vi "Save_Raw_data.vi"(4 "Add to Block Header":string, 7 "append to file? (new file:F)":bool, 8 "Block Timings":T1) -> (2 "Block Header":string)   [LabVIEW 2017]
uses:
  Controls/Block_start_and_end.ctl
  Globals/LDA_meas_global_1.vi
  Globals/LDA_meas_global_2.vi
  Acquisition/PWA/PWAtasksGLOBAL.vi
  Globals/Meas_global.vi
  Globals/Constants_global.vi
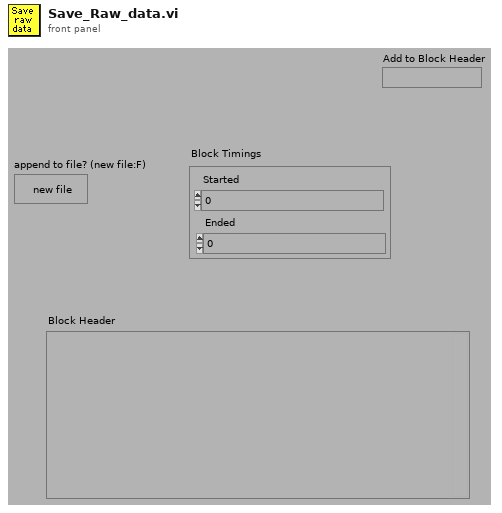
[diagram p1: front panel]
types:
  T1 = typedef "Block_start_and_end.ctl" = cluster{"Started":dbl, "Ended":dbl}
  T2 = typedef "BSA_Type.ctl" = enum16{"57N11", "BSA F60"}
  T3 = cluster{"scale multiplier":dbl, "scale offset":dbl, "Length":i32, "I16 data":i16[], "Sampling rate (Hz)":dbl}
  T4 = typedef "Analysis_info_cluster.ctl" = cluster{"Colour":u32, "Inst type":T5, "Inst name":string, "Symbol":string, "Code name":string, "Extra Info":string, "Inst Array":T6, "Extra Titles":string[], "Extra Values":string[], "U":dbl, "u^2":dbl, "u^3":dbl, "u^4":dbl, "Skew_u":dbl, "Kurt_u":dbl, "Sd Error in Mean":dbl, "% u'/U":dbl, "X":dbl, "Y":dbl, "Z":dbl, "Timescale integral Estimate":dbl, "Sd Error in Variance":dbl, "Calib File":path, "Calib Constants":dbl[], "Output Position":bool, "Full Stats":bool, "Av Sampling Rate":dbl, "Av No of Samples":dbl, "Total Meas Time (s)":dbl, "ADAM Ch Name":string, "Max value":dbl, "Min value":dbl, "Sync Delay Time (s)":dbl}
  T5 = typedef "Inst_type.ctl" = enum16{"Propeller anemometer", "Raw voltage", "Pressure Transducer", "Pitot-static tube", "Preston tube", "Hot wire", "Cross wire 1", "Cross wire 2", "Generic Linear", "Generic Polynomial", "Generic BackPoly", "Fast FID", "Thermocouple", "Cold wire", "Pulsed Wire", "LDA Vel", "LDA Tran time", "LDA Arr time", "Microphone"}
  T6 = typedef "Instrument_Array.ctl" = enum16{"PWA", "LDA", "Analogue"}
  T7 = typedef "Time_Trace_Cluster.ctl" = cluster{"Weighting":dbl[], "Time (s)":dbl[], "Voltage":dbl[], "Eng Values":dbl[]}
  T8 = cluster{"scale multiplier":dbl, "scale offset":dbl}[]
  T9 = typedef "PWA_Data.ctl" = enum16{"No PWA Data", "One Ch PWA"}
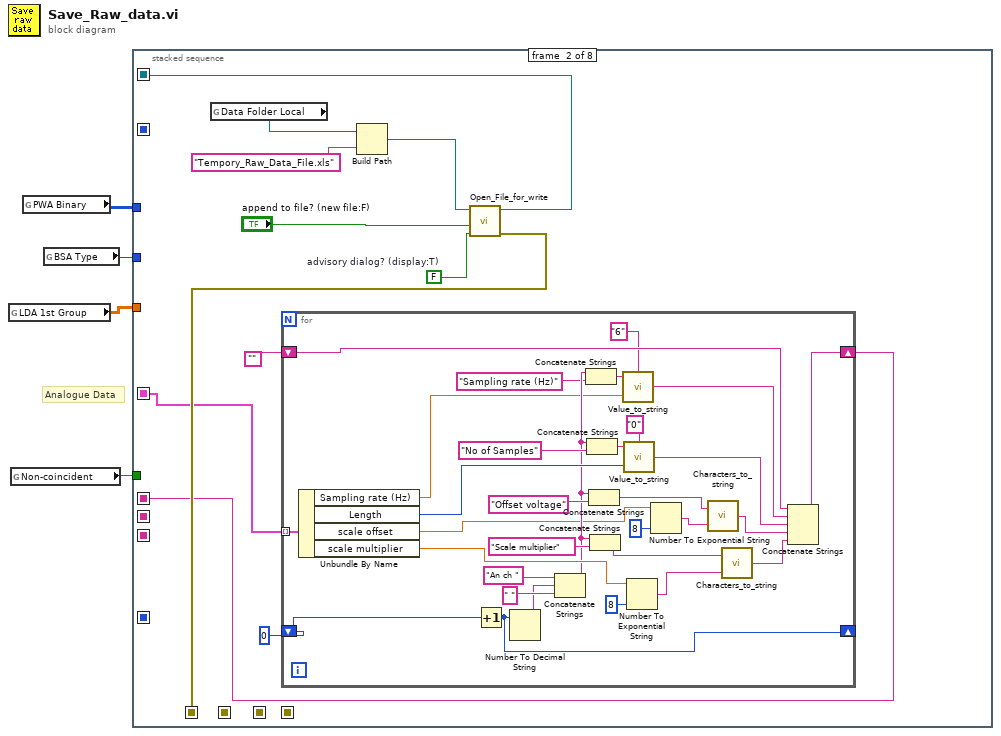
[diagram p0: block diagram]
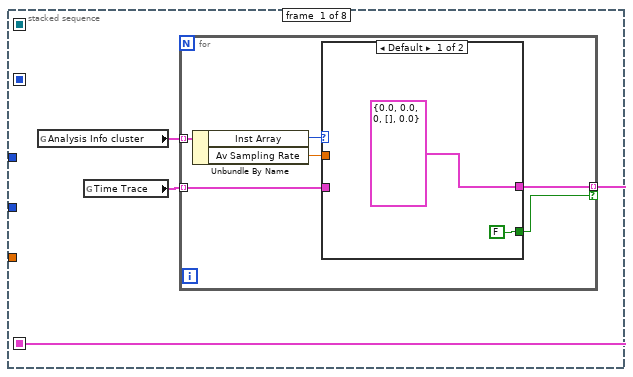
[diagram p2: hidden frame]
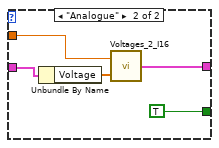
[diagram p3: hidden frame]
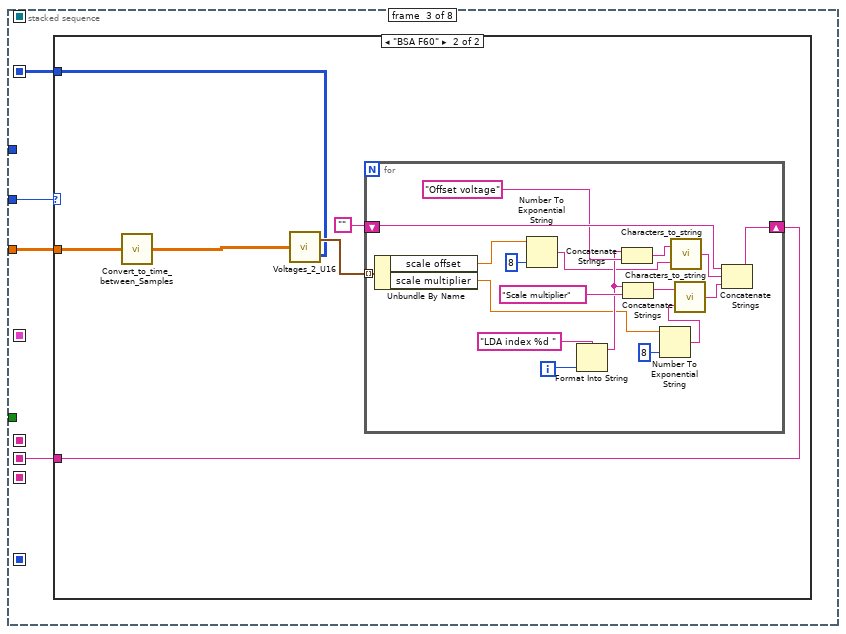
[diagram p4: hidden frame]
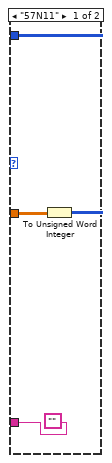
[diagram p5: hidden frame]
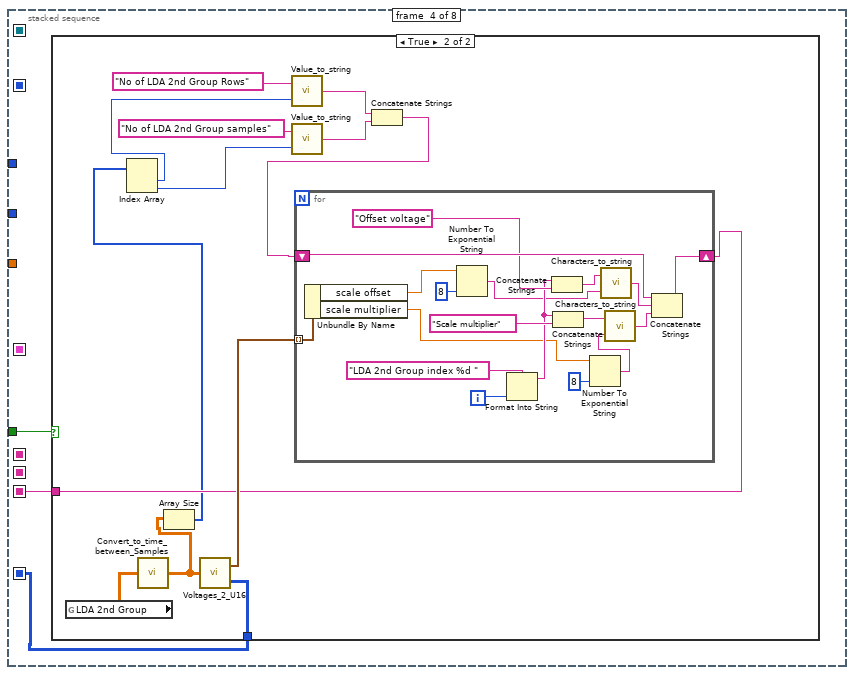
[diagram p6: hidden frame]
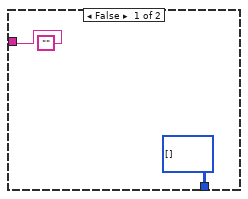
[diagram p7: hidden frame]
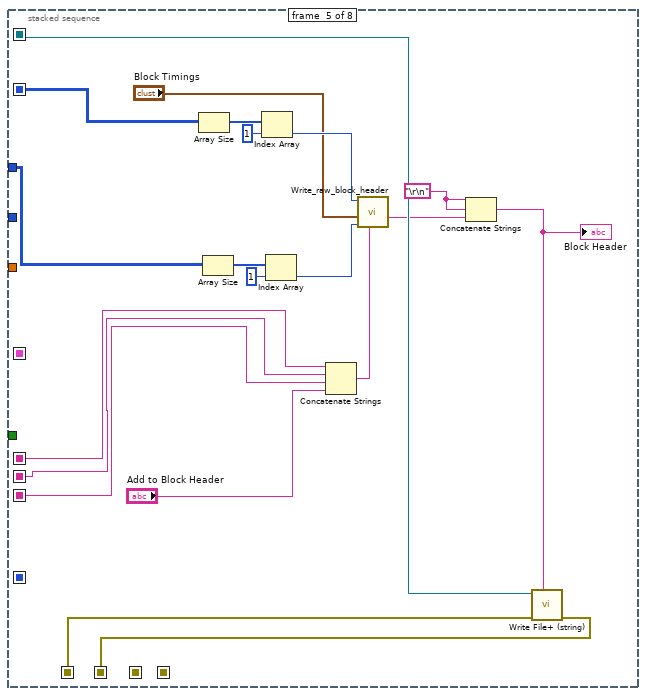
[diagram p8: hidden frame]
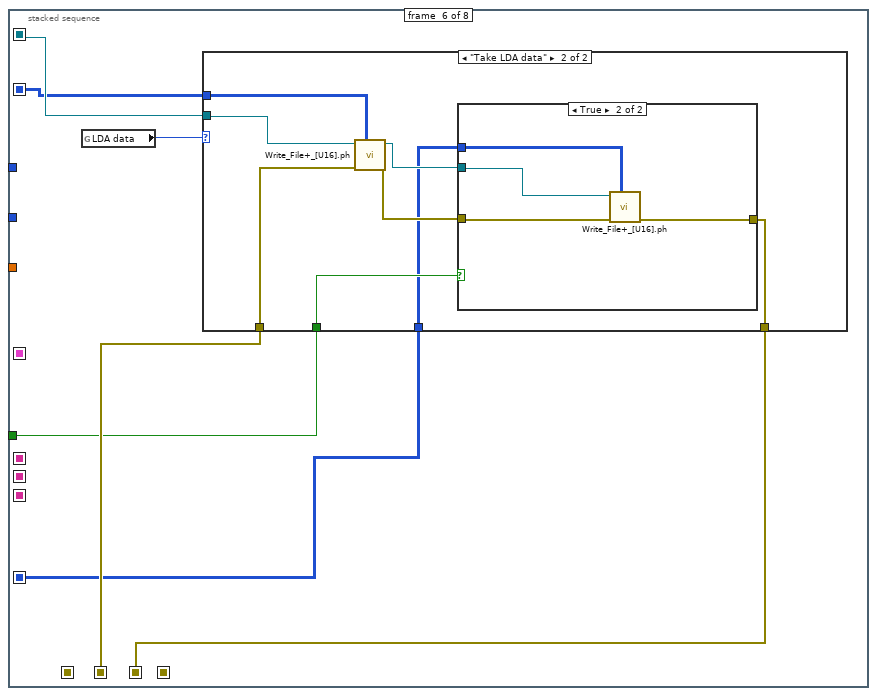
[diagram p9: hidden frame]
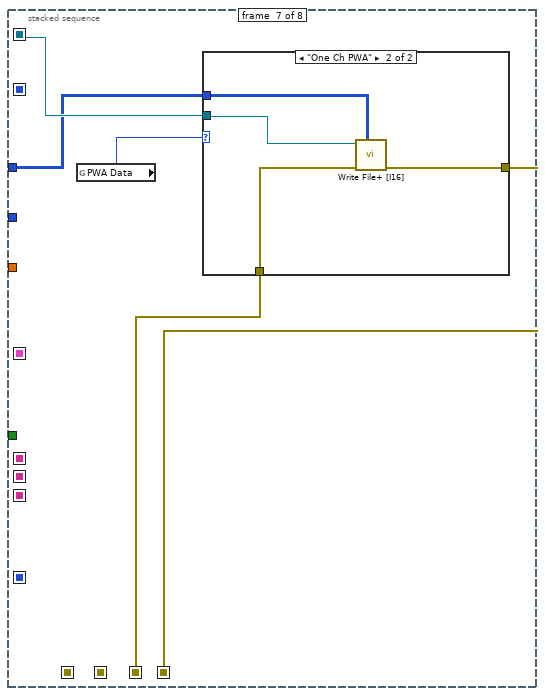
[diagram p12: hidden frame]
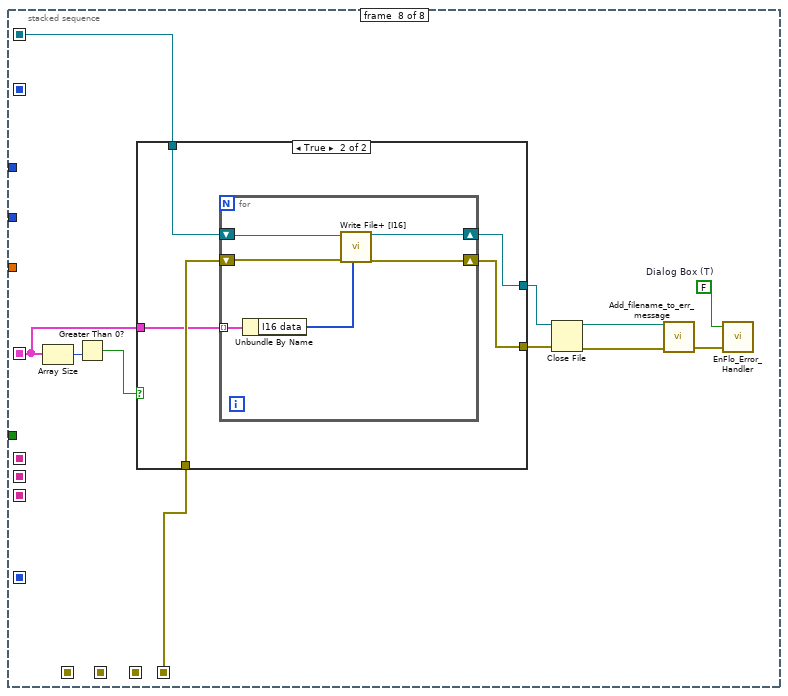
[diagram p14: hidden frame]
diagram:
  # "Analogue Data"
  n1 = global read "LDA_meas_global_2.vi" "LDA 1st Group"() -> (w2:dbl[][])
  n2 = global read "LDA_meas_global_1.vi" "Non-coincident"() -> (w4:bool)
  n3 = global read "PWAtasksGLOBAL.vi" "PWA Binary"() -> (w1:i16[][])
  n4 = global read "LDA_meas_global_1.vi" "BSA Type"() -> (w3:T2)
  n5 = stacked-sequence {
    seq-local: [_ w31 _ _ _ _ _ _] -> [_ _ _ _ w146 w154 w174 w191]
    seq-local: [_ w30 _ _ _ _ _ _] -> [_ _ _ _ w145 _ _ _]
    seq-local: [_ _ _ _ w144 _ _ _] -> [_ _ _ _ _ w155 _ _]
    seq-local: [_ _ _ _ _ w151 _ _] -> [_ _ _ _ _ _ w173 _]
    seq-local: [_ _ _ _ _ _ w172 _] -> [_ _ _ _ _ _ _ w184]
    seq-local: [_ _ _ w96 _ _ _ _] -> [_ _ _ _ _ w152 _ _]
    seq-local: [_ _ _ w94 _ _ _ _] -> [_ _ _ _ w134 _ _ _]
    seq-local: [_ w22 _ _ _ _ _ _] -> [_ _ _ _ w132 _ _ _]
    seq-local: [_ _ w64 _ _ _ _ _] -> [_ _ _ _ w130 w150 _ _]
    seq-local: [_ _ w63 _ _ _ _ _] -> [_ _ _ _ w131 _ _ _]
    seq-local: [w5 _ _ _ _ _ _ _] -> [_ w21 _ _ _ _ _ w181]
    tunnel: w1 -> [_ _ _ _ w138 _ w171 _]
    tunnel: w4 -> [_ _ _ w95 _ w153 _ _]
    tunnel: w3 -> [_ _ w66 _ _ _ _ _]
    tunnel: w2 -> [_ _ w65 _ _ _ _ _]
    frame #0 {
      n6 = global read "Meas_global.vi" "Analysis Info cluster"() -> (w7:T4[])
      n7 = global read "Meas_global.vi" "Time Trace"() -> (w6:T7[])
      n8 = for {
        tunnel: w7 -> [w13] mode=indexing
        tunnel: w6 -> [w11] mode=indexing
        tunnel: [w10] -> w5 mode=indexing if=w9
        n9 = Unbundle By Name(w13) -> ("Inst Array"=w12:T6, "Av Sampling Rate"=w8:dbl)
        n10 = case shown="Default" w12 {
          tunnel: w11 -> [_ w20]
          tunnel: [T3 {"scale multiplier"=0.0, "scale offset"=0.0, "Length"=0, "I16 data"=[], "Sampling rate (Hz)"=0.0} ("Channel Data") w16] -> w10
          tunnel: [FALSE TRUE] -> w9
          tunnel: w8 -> [_ w17]
          frame Default {
          }
          frame "Analogue" {
            n11 = Unbundle By Name(w20) -> ("Voltage"=w19:dbl[])
            n12 = call "Voltages_2_I16.vi"("Voltages"=w19, "Av Sampling Rate"=w17) -> ("Channel Data"=w16:T3)
          }
        }
      }
    }
    frame #1 {
      w29 = FALSE  # advisory dialog? (display:T)
      n13 = global read "Constants_global.vi" "Data Folder Local"() -> (w28:path)
      n14 = for {
        shift-right: [w62] -> w22
        shift-left: "" -> [w40]
        shift-right: [w60] -> _
        shift-left: 0 -> [w61]
        tunnel: w21 -> [w50] mode=indexing
        n15 = Unbundle By Name(w50) -> ("Sampling rate (Hz)"=w41:dbl, "Length"=w46:i32, "scale offset"=w34:dbl, "scale multiplier"=w49:dbl)
        n16 = Increment(x=w61) -> (x+1=w60:i32)
        n17 = Number To Decimal String(number=w60) -> (decimal integer string=w55:string)  [unwired: 1 out]
        n18 = Concatenate Strings("An ch ", w55, " ") -> (w43:string)
        n19 = Concatenate Strings(w43, "Sampling rate (Hz)" ("string")) -> (w44:string)
        n20 = Concatenate Strings(w43, "No of Samples") -> (w48:string)
        n21 = Concatenate Strings(w43, "Offset voltage") -> (w35:string)
        n22 = Concatenate Strings(w43, "Scale multiplier") -> (w52:string)
        n23 = call "Value_to_string.vi"("precision"="6", "Value"=w41, "Label for value"=w44) -> ("Output string"=w39:string)
        n24 = call "Value_to_string.vi"("precision"="0", "Value"=w46, "Label for value"=w48) -> ("Output string"=w38:string)
        n25 = Number To Exponential String(number=w49, precision (6)=i16 8) -> (E-format string=w51:string)  [unwired: 2 out]
        n26 = Number To Exponential String(number=w34, precision (6)=i16 8) -> (E-format string=w36:string)  [unwired: 2 out]
        n27 = call "Characters_to_string.vi"("Characters to write"=w36, "Label for characters"=w35) -> ("Output string"=w33:string)
        n28 = call "Characters_to_string.vi"("Characters to write"=w51, "Label for characters"=w52) -> ("Output string"=w53:string)
        n29 = Concatenate Strings(w40, w39, w38, w33, w53) -> (w62:string)
      }
      n30 = Build Path(base path=w28, name or relative path="Tempory_Raw_Data_File.xls") -> (appended path=w26:path)
      n31 = call "Open_File_for_write.vi"("advisory dialog? (display:T)"=w29, "append to file? (new file:F)"="append to file? (new file:F)", "file path"=w26) -> ("error out"=w30:errorcluster, "refnum"=w31:refnum<file>)  [unwired: 7 out]
    }
    frame #2 {
      n32 = case shown="\"BSA F60\"" w66 {
        tunnel: w65 -> [w69 w71]
        tunnel: [w68 w74] -> w64
        tunnel: ["" w73] -> w63
        frame "57N11" {
          n33 = To Unsigned Word Integer(number=w69) -> (unsigned 16bit integer=w68:u16[][])
        }
        frame "BSA F60" {
          n34 = call "Convert_to_time_between_Samples.vi"("LDA 1st Group in"=w71) -> ("LDA 1st Group out"=w70:dbl[][])
          n35 = call "Voltages_2_U16.vi"("Voltages"=w70) -> ("Scale and Offset"=w75:T8, "U16 data"=w74:u16[][])
          n36 = for {
            shift-right: [w92] -> w73
            shift-left: "" -> [w93]
            tunnel: w75 -> [w85] mode=indexing
            i -> [w82]
            n37 = Unbundle By Name(w85) -> ("scale offset"=w78:dbl, "scale multiplier"=w81:dbl)
            n38 = Number To Exponential String(number=w78, precision (6)=i16 8) -> (E-format string=w77:string)  [unwired: 2 out]
            n39 = Format Into String(format string="LDA index %d ", w82) -> (resulting string=w83:string)  [unwired: 2 in, 1 out]
            n40 = Concatenate Strings(w83, "Offset voltage") -> (w80:string)
            n41 = Concatenate Strings(w83, "Scale multiplier") -> (w87:string)
            n42 = Number To Exponential String(number=w81, precision (6)=i16 8) -> (E-format string=w86:string)  [unwired: 2 out]
            n43 = call "Characters_to_string.vi"("Characters to write"=w77, "Label for characters"=w80) -> ("Output string"=w76:string)
            n44 = call "Characters_to_string.vi"("Characters to write"=w86, "Label for characters"=w87) -> ("Output string"=w88:string)
            n45 = Concatenate Strings(w93, w76, w88) -> (w92:string)
          }
        }
      }
    }
    frame #3 {
      n46 = case shown="True" w95 {
        tunnel: [u16[][] [] ("U16 data") w111] -> w96
        tunnel: ["" w109] -> w94
        frame False {
        }
        frame True {
          n47 = global read "LDA_meas_global_2.vi" "LDA 2nd Group"() -> (w100:dbl[][])
          n48 = call "Convert_to_time_between_Samples.vi"("LDA 1st Group in"=w100) -> ("LDA 1st Group out"=w99:dbl[][])
          n49 = Array Size(array=w99) -> (size(s)=w106:i32[])
          n50 = Index Array(array=w106) -> (element #1=w105:i32, element #2=w104:i32)  [unwired: 2 in]
          n51 = call "Voltages_2_U16.vi"("Voltages"=w99) -> ("Scale and Offset"=w110:T8, "U16 data"=w111:u16[][])
          n52 = call "Value_to_string.vi"("Value"=w105, "Label for value"="No of LDA 2nd Group Rows") -> ("Output string"=w103:string)  [unwired: 1 in]
          n53 = call "Value_to_string.vi"("Value"=w104, "Label for value"="No of LDA 2nd Group samples") -> ("Output string"=w102:string)  [unwired: 1 in]
          n54 = Concatenate Strings(w103, w102) -> (w101:string)
          n55 = for {
            shift-right: [w128] -> w109
            shift-left: w101 -> [w129]
            tunnel: w110 -> [w121] mode=indexing
            i -> [w118]
            n56 = Unbundle By Name(w121) -> ("scale offset"=w114:dbl, "scale multiplier"=w117:dbl)
            n57 = Number To Exponential String(number=w114, precision (6)=i16 8) -> (E-format string=w113:string)  [unwired: 2 out]
            n58 = Format Into String(format string="LDA 2nd Group index %d ", w118) -> (resulting string=w119:string)  [unwired: 2 in, 1 out]
            n59 = Concatenate Strings(w119, "Offset voltage") -> (w116:string)
            n60 = Concatenate Strings(w119, "Scale multiplier") -> (w123:string)
            n61 = Number To Exponential String(number=w117, precision (6)=i16 8) -> (E-format string=w122:string)  [unwired: 2 out]
            n62 = call "Characters_to_string.vi"("Characters to write"=w113, "Label for characters"=w116) -> ("Output string"=w112:string)
            n63 = call "Characters_to_string.vi"("Characters to write"=w122, "Label for characters"=w123) -> ("Output string"=w124:string)
            n64 = Concatenate Strings(w129, w112, w124) -> (w128:string)
          }
        }
      }
    }
    frame #4 {
      w141 = "\r\n"
      n65 = Array Size(array=w130) -> (size(s)=w148:i32[])
      n66 = Array Size(array=w138) -> (size(s)=w139:i32[])
      n67 = Index Array(array=w148, index=1) -> (element=w147:i32)
      n68 = Index Array(array=w139, index=1) -> (element=w137:i32)
      n69 = Concatenate Strings(w132, w131, w134, "Add to Block Header") -> (w133:string)
      n70 = call "Write_raw_block_header.vi"("No of LDA samples"=w147, "Block Timings"="Block Timings", "No of PWA samples"=w137, "Add to Block Header"=w133) -> ("Output string"=w142:string)  [unwired: 1 in]
      n71 = Concatenate Strings(w141, w141, w142) -> (w136:string)
      "Block Header" <- w136
      n72 = call <vilib>:"Write File+ (string).vi"("string"=w136, "error in (no error)"=w145, "refnum"=w146) -> ("error out"=w144:errorcluster)  [unwired: 2 in, 4 out]
    }
    frame #5 {
      n73 = global read "Meas_global.vi" "LDA data"() -> (w156:enum16{"No LDA data", "Take LDA data"})
      n74 = case shown="\"Take LDA data\"" w156 {
        tunnel: w150 -> [_ w165]
        tunnel: w154 -> [_ w164]
        tunnel: w155 -> [w157 w163]
        tunnel: w153 -> [_ w162]
        tunnel: w152 -> [_ w158]
        tunnel: [w157 w159] -> w151
        frame "No LDA data" {
        }
        frame "Take LDA data" {
          n75 = call "Write_File+_[U16].ph.vi"("2D array"=w165, "error in (no error)"=w163, "refnum"=w164) -> ("error out"=w160:errorcluster, "dup refnum"=w161:refnum<file>)  [unwired: 3 in, 4 out]
          n76 = case shown="True" w162 {
            tunnel: w158 -> [_ w170]
            tunnel: w161 -> [_ w169]
            tunnel: [w166 w168] -> w159
            tunnel: w160 -> [w166 w167]
            frame False {
            }
            frame True {
              n77 = call "Write_File+_[U16].ph.vi"("2D array"=w170, "error in (no error)"=w167, "refnum"=w169) -> ("error out"=w168:errorcluster)  [unwired: 3 in, 5 out]
            }
          }
        }
      }
    }
    frame #6 {
      n78 = global read "Meas_global.vi" "PWA Data"() -> (w175:T9)
      n79 = case shown="\"One Ch PWA\"" w175 {
        tunnel: w171 -> [_ w178]
        tunnel: w174 -> [_ w177]
        tunnel: w173 -> [w176 w180]
        tunnel: [w176 w179] -> w172
        frame "No PWA Data" {
        }
        frame "One Ch PWA" {
          n80 = call <vilib>:"Write File+ [I16].vi"("2D array"=w178, "error in (no error)"=w180, "refnum"=w177) -> ("error out"=w179:errorcluster)  [unwired: 3 in, 5 out]
        }
      }
    }
    frame #7 {
      w189 = FALSE  # Dialog Box (T)
      n81 = Array Size(array=w181) -> (size(s)=w183:i32)
      n82 = Greater Than 0?(x=w183) -> (x > 0?=w182:bool)
      n83 = case shown="True" w182 {
        tunnel: w191 -> [w193 w195]
        tunnel: w184 -> [w192 w198]
        tunnel: [w192 w197] -> w188
        tunnel: [w193 w196] -> w187
        tunnel: w181 -> [_ w194]
        frame False {
        }
        frame True {
          n84 = for {
            shift-right: [w203] -> w197
            shift-left: w198 -> [w204]
            shift-right: [w202] -> w196
            shift-left: w195 -> [w201]
            tunnel: w194 -> [w200] mode=indexing
            n85 = Unbundle By Name(w200) -> ("I16 data"=w199:i16[])
            n86 = call <vilib>:"Write File+ [I16].vi"("1D array"=w199, "error in (no error)"=w204, "refnum"=w201) -> ("error out"=w203:errorcluster, "dup refnum"=w202:refnum<file>)  [unwired: 3 in, 4 out]
          }
        }
      }
      n87 = Close File(refnum=w187, error in=w188) -> (path=w185:path, error out=w186:errorcluster)
      n88 = call "Add_filename_to_err_message.vi"("error in (no error)"=w186, "Path"=w185) -> ("error out"=w190:errorcluster)
      n89 = call "EnFlo_Error_Handler.vi"("error in (no error)"=w190, "Dialog Box (T)"=w189) -> ()  [unwired: 1 in, 3 out]
    }
  }
